vi "TestSilentVS.vi"() -> ()   [LabVIEW 2011]
uses:
  <vilib>/NI Veristand/Execution/ModelManager/NI VeriStand - Set Single Parameter Value.vi
  <vilib>/NI Veristand/Execution/ModelManager/NI VeriStand - Get Single Parameter Value.vi
  <vilib>/NI Veristand/Execution/Workspace/NI_VS Workspace ExecutionAPI.lvlib
  <vilib>/NI Veristand/Execution/ModelManager/NI_VS ModelManager ExecutionAPI.lvlib
panel:
  in  "systemdefintion_file_path":path=path "C:/Users/Public/Documents/National Instruments/NI VeriStand 2011/Projects/Example/Sinewave Delay.nivssdf"
  out "Parameters":string[](array[string])
  out "Value":dbl
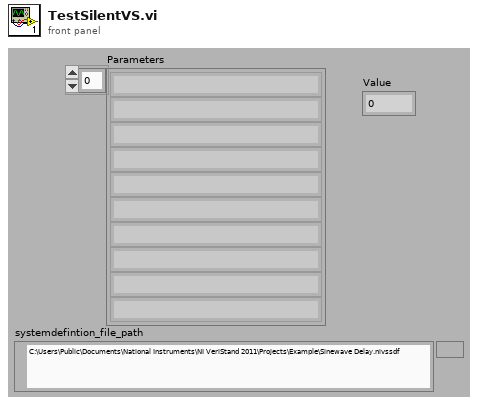
[diagram p1: front panel]
types:
  T1 = typedef "NI_VS Workspace ExecutionAPI.lvlib/WorkspaceAPI.ctl" = refnum<k24>
  T2 = typedef "NI_VS ModelManager ExecutionAPI.lvlib/ModelManagerAPI.ctl" = refnum<k24>
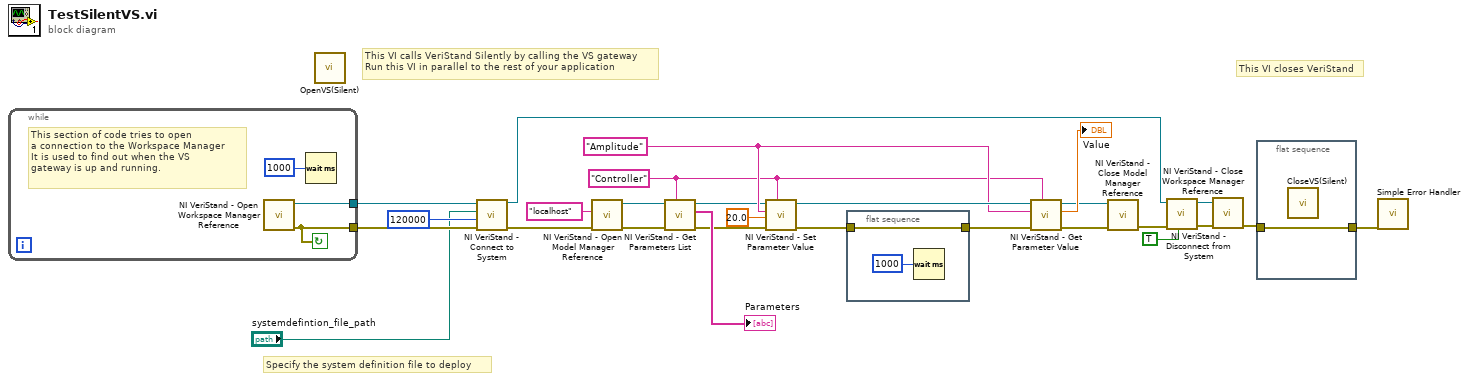
[diagram p0: block diagram]
diagram:
  w16 = "Controller" ("Target")
  w23 = "Amplitude" ("Parameter")
  # "Specify the system definition file to deploy"
  # "This VI closes VeriStand"
  # "This VI calls VeriStand Silently by calling the VS gateway\nRun this VI in parallel to the rest of your application"
  n1 = while {
    tunnel: [w29] -> w12
    tunnel: [w28] -> w14
    stop <- w28 continue-if-true
    # "This section of code tries to open \na connection to the Workspace Manager\nIt is used to find out when the VS\ngateway is up and running."
    n2 = call <vilib>:"NI VeriStand - Open Workspace Manager Reference.vi"() -> ("error out"=w28:errorcluster, "WorkspaceManager"=w29:T1)  [unwired: 10 in]
    n3 = Wait (ms)(milliseconds to wait=u32 1000) -> ()  [unwired: 1 out]
  }
  n4 = call "OpenVS(Silent).vi"() -> ()  [unwired: 12 in]
  n5 = call <vilib>:"NI VeriStand - Connect to System.vi"("error in (no error)"=w14, "Timeout (60000 ms)"=u32 120000, "System Definition File (.nivssdf)"="systemdefintion_file_path", "WorkspaceManager in"=w12) -> ("error out"=w13:errorcluster, "WorkspaceManager out"=w4:T1)  [unwired: 6 in]
  n6 = call <vilib>:"NI VeriStand - Open Model Manager Reference.vi"("error in (no error)"=w13, "Gateway IP Address (\"\": localhost)"="localhost" ("Gateway IP Address (\"\": localhost)")) -> ("error out"=w19:errorcluster, "ModelManager"=w21:T2)  [unwired: 8 in]
  n7 = call <vilib>:"NI VeriStand - Get Parameters List.vi"("Target"=w16, "error in (no error)"=w19, "ModelManager in"=w21) -> ("error out"=w18:errorcluster, "Parameters"=→"Parameters":string[], "ModelManager out"=w17:T2)  [unwired: 6 in]
  n8 = call-poly <vilib>:"NI VeriStand - Set Parameter Value.vi"("Target"=w16, "error in (no error)"=w18, "Value"=20.0, "Parameter"=w23, "ModelManager in"=w17) -> ("error out"=w26:errorcluster, "ModelManager out"=w24:T2)  [unwired: 5 in]
  n9 = flat-sequence {
    tunnel: w26 -> [w31]
    tunnel: [w31] -> w25
    frame #0 {
      n10 = Wait (ms)(milliseconds to wait=u32 1000) -> ()  [unwired: 1 out]
    }
  }
  n11 = call-poly <vilib>:"NI VeriStand - Get Parameter Value.vi"("Target"=w16, "error in (no error)"=w25, "Parameter"=w23, "ModelManager in"=w24) -> ("error out"=w8:errorcluster, "Value"=→"Value":dbl, "ModelManager out"=w7:T2)  [unwired: 5 in]
  n12 = call <vilib>:"NI VeriStand - Close Model Manager Reference.vi"("error in (no error)"=w8, "ModelManager"=w7) -> ("error out"=w6:errorcluster)  [unwired: 9 in]
  n13 = call <vilib>:"NI VeriStand - Disconnect from System.vi"("Undeploy System Definition (F)"=TRUE, "error in (no error)"=w6, "WorkspaceManager in"=w4) -> ("error out"=w3:errorcluster, "WorkspaceManager out"=w2:T1)  [unwired: 7 in]
  n14 = call <vilib>:"NI VeriStand - Close Workspace Manager Reference.vi"("error in (no error)"=w3, "WorkspaceManager"=w2) -> ("error out"=w1:errorcluster)  [unwired: 9 in]
  n15 = flat-sequence {
    tunnel: w1 -> [w33]
    tunnel: [w33] -> w15
    frame #0 {
      n16 = call "CloseVS(Silent).vi"() -> ()  [unwired: 12 in]
    }
  }
  n17 = call <vilib>:"Simple Error Handler.vi"("error in (no error)"=w15) -> ()  [unwired: 4 in, 5 out]
